vi "1_07.vi"() -> ()   [LabVIEW 2018]
uses:
  <vilib>/sound2/lvsound2.llb/Sound Data Format.ctl
  <vilib>/sound2/lvsound2.llb/Sound Output Write (DBL).vi
  <vilib>/measure/NI_MABase.lvlib
panel:
  in  "Frecuencia 2":dbl
  in  "Amplitud 2":dbl
  in  "Frecuencia":dbl
  in  "Amplitud":dbl
  in  "stop":bool
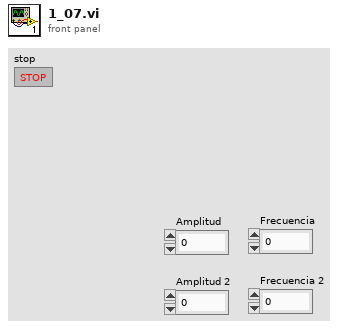
[diagram p1: front panel]
types:
  T1 = typedef "Sound Data Format.ctl" = cluster{"sample rate (S/s)":dbl, "number of channels":i32, "bits per sample":i32}
  T2 = typedef "Sound Output Task ID.ctl" = u32
  T3 = cluster{"sample rate (S/s)":dbl, "number of samples/ch":i32}
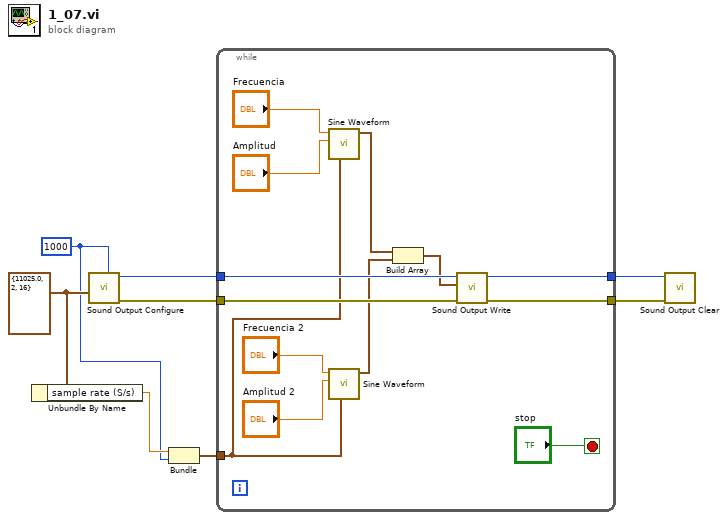
[diagram p0: block diagram]
diagram:
  w2 = 1000 ("number of samples/ch")
  w4 = T1 {"sample rate (S/s)"=11025.0, "number of channels"=2, "bits per sample"=16} ("sound format")
  n1 = Unbundle By Name(w4) -> ("sample rate (S/s)"=w3:dbl)
  n2 = call <vilib>:"Sound Output Configure.vi"("number of samples/ch"=w2, "sound format"=w4) -> ("error out"=w7:errorcluster, "task ID"=w8:T2)  [unwired: 8 in]
  n3 = Bundle("sample rate (S/s)"=w3, "number of samples/ch"=w2) -> (w1:T3)  [unwired: 1 in]
  n4 = while {
    tunnel: w8 -> [w20]
    tunnel: w7 -> [w19]
    tunnel: [w18] -> w6
    tunnel: [w17] -> w5
    tunnel: w1 -> [w12]
    stop <- "stop" stop-if-true
    n5 = call <vilib>:"Sine Waveform.vi"("sampling info"=w12, "amplitude"="Amplitud", "frequency"="Frecuencia") -> ("signal out"=w11:waveform(dbl))  [unwired: 7 in, 1 out]
    n6 = call <vilib>:"Sine Waveform.vi"("sampling info"=w12, "amplitude"="Amplitud 2", "frequency"="Frecuencia 2") -> ("signal out"=w10:waveform(dbl))  [unwired: 7 in, 1 out]
    n7 = Build Array(w11, w10) -> (w9:waveform(dbl)[])
    n8 = call-poly <vilib>:"Sound Output Write.vi"("error in (no error)"=w19, "data"=w9, "task ID"=w20) -> ("error out"=w17:errorcluster, "task ID out"=w18:T2)  [unwired: 7 in]
  }
  n9 = call <vilib>:"Sound Output Clear.vi"("error in (no error)"=w5, "task ID"=w6) -> ()  [unwired: 9 in, 1 out]
